vi "HistoryGraph.vi"() -> ()   [LabVIEW 2016, in "PCM MenuVIPanelSplit.lvclass"]
uses:
  PCM MenuVIPanelSplit.lvclass
  PanelSplitToolkit/PanelObject/PanelObject.lvclass
  PanelSplitToolkit/QueueManager.llb/Remove.vi
  <vilib>/Utility/error.llb/DialogType.ctl
  PanelSplitToolkit/PanelDataNode/PanelDataNode.lvclass
  PanelSplitToolkit/QueueManager.llb/Insert.vi
  PanelSplitToolkit/QueueManager.llb/CreatQueue.vi
  PanelSplitToolkit/QueueManager.llb/Destroy.vi
  <vilib>/measure/NI_MAPro.lvlib
  <vilib>/measure/maspectr.llb/FFT Spectrum (Mag-Phase) for 1 Chan.vi
  <vilib>/measure/maspectr.llb/FFT Power Spectrum and PSD for 1 Chan.vi
  <vilib>/measure/NI_MABase.lvlib
  <vilib>/Analysis/4window.llb/windowTd.ctl
  <vilib>/Analysis/NI_AALPro.lvlib
  Display Mode.ctl
  PCM PanelSplit.lvclass
  Display Config.ctl
  <vilib>/Utility/miscctls.llb/LVRangeTypeDef.ctl
panel:
  in  "Node*":refnum<data-value>
  out "波形图":waveform(dbl)[](graph)
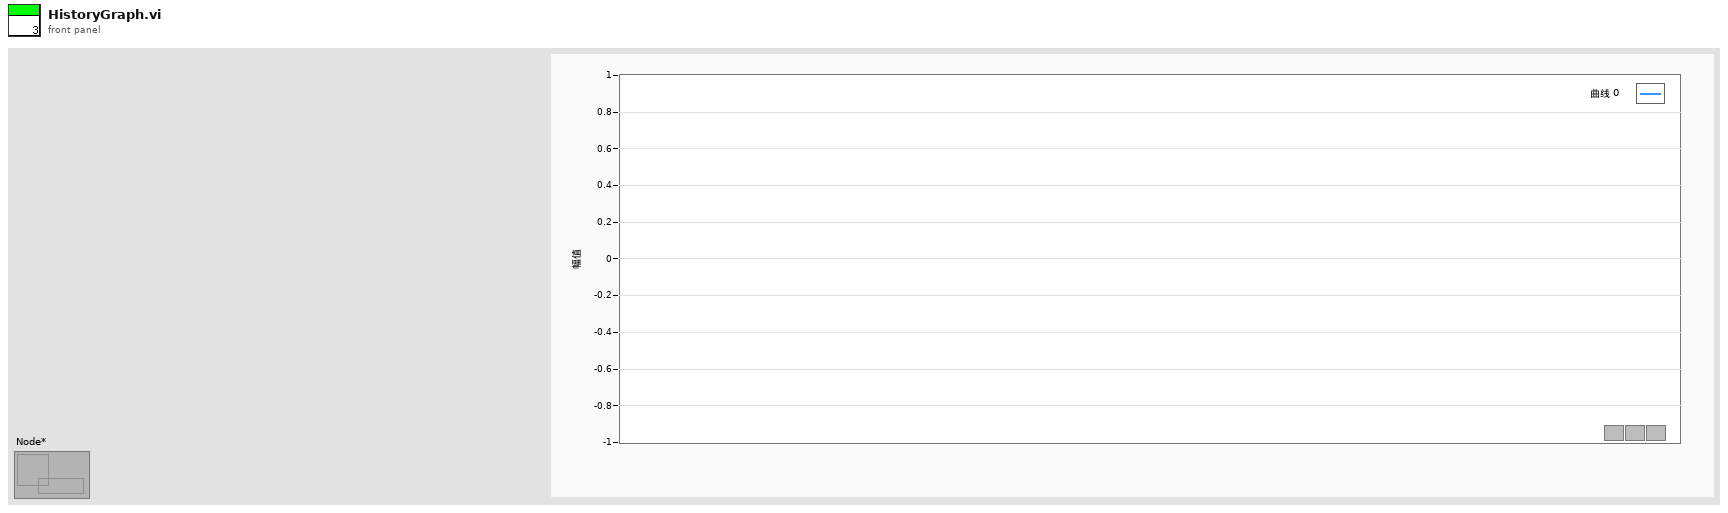
[diagram p1: front panel]
types:
  T1 = cluster{"Name":string, "Color":u32, "Style":u8, "Point Style":u8, "Name Visible":bool, "Allow Drag":bool, "Annotation Mode":u32, "Plot":i32, "Index":i32, "Position":cluster{"X":dbl, "Y":dbl}, "X Scale":u32, "Y Scale":u32, "Show Arrow":bool, "Lock Name":bool, "Plot Area":i32, "Label Offset":cluster{"X":dbl, "Y":dbl}}
  T2 = typedef "PCM PanelSplit.lvclass/Display Config.ctl" = cluster{"Display Mode":T3, "ChTag[]":string[], "window":T4, "Range":T5}
  T3 = typedef "PCM PanelSplit.lvclass/Display Mode.ctl" = enum16{"时域", "频谱", "功率谱"}
  T4 = typedef "NI_AALPro.lvlib/windowTd.ctl" = u32
  T5 = typedef "LVRangeTypeDef.ctl" = cluster{"Minimum":dbl, "Maximum":dbl, "Increment":dbl, "Minor Increment":dbl, "Start":dbl}
  T6 = cluster{"error":errorcluster, "LocalQ":cluster{"LQName":string, "LQEvent":string, "LQData":variant}, "HighQ":cluster{"HQName":string, "HQEvent":string, "HQData":variant}, "Display Config":T2, "波形图表":refnum<vi>, "波形图":refnum<vi>}
  T7 = typedef "DialogType.ctl" = u16
  T8 = typedef "Analysis Parameters.ctl" = cluster{"Enable":cluster{"Wave":bool, "Filter":bool, "FFT":bool, "Power":bool, "Shock":bool}, "IIR Parameter":T9, "FFT Parameters":T10, "Power Parameters":T12, "Shock Parameter ":T13}
  T9 = typedef "IIR Parameter.ctl" = cluster{"Filter Type":u16, "Filter Topology":u16, "Order":u32, "Lower Cut-Off":dbl, "Upper Cut-Off":dbl}
  T10 = typedef "FFT Parameters.ctl" = cluster{"window":T11, "frequency range":cluster{"start frequency":dbl, "stop frequency":dbl}, "view":cluster{"dB On (T)":bool, "unwrap phase (F)":bool, "convert to degree (T)":bool}, "averaging parameters":cluster{"averaging mode":enum16{"No averaging", "Vector averaging", "RMS averaging", "Peak hold"}, "weighting mode":enum16{"Linear", "Exponential"}, "number of averages":u32, "linear mode":enum16{"One shot", "Auto restart"}}}
  T11 = typedef "svc_Window.ctl" = u32
  T12 = typedef "Power Parameters.ctl" = cluster{"window":T11, "frequency range":cluster{"start frequency":dbl, "stop frequency":dbl}, "dB On (T)":bool, "averaging parameters":cluster{"averaging mode":enum16{"No averaging", "Vector averaging", "RMS averaging", "Peak hold"}, "weighting mode":enum16{"Linear", "Exponential"}, "number of averages":u32, "linear mode":enum16{"One shot", "Auto restart"}}}
  T13 = typedef "Shock Parameter.ctl" = cluster{"frequency range":cluster{"low frequency [Hz]":dbl, "high frequency [Hz]":dbl, "frequencies / octave":i32}, "model":i32, "critical damping factor":dbl, "preprocessing settings":cluster{"lowpass filter On ? (F)":bool, "lowpass cutoff frequency [Hz]":dbl, "remove DC ? (F)":bool}, "displacement units":i32, "maximum value type":i32, "pulse duration [ms]":dbl}
  T14 = cluster{"Name":string, "Color":u32, "Style":u8, "Point Style":u8, "Name Visible":bool, "Allow Drag":bool, "Annotation Mode":u32, "Plot":i32, "Index":i32, "Position":cluster{"X":dbl, "Y":dbl}, "X Scale":u32, "Y Scale":u32, "Show Arrow":bool, "Lock Name":bool, "Plot Area":i32, "Label Offset":cluster{"X":dbl, "Y":dbl}}[]
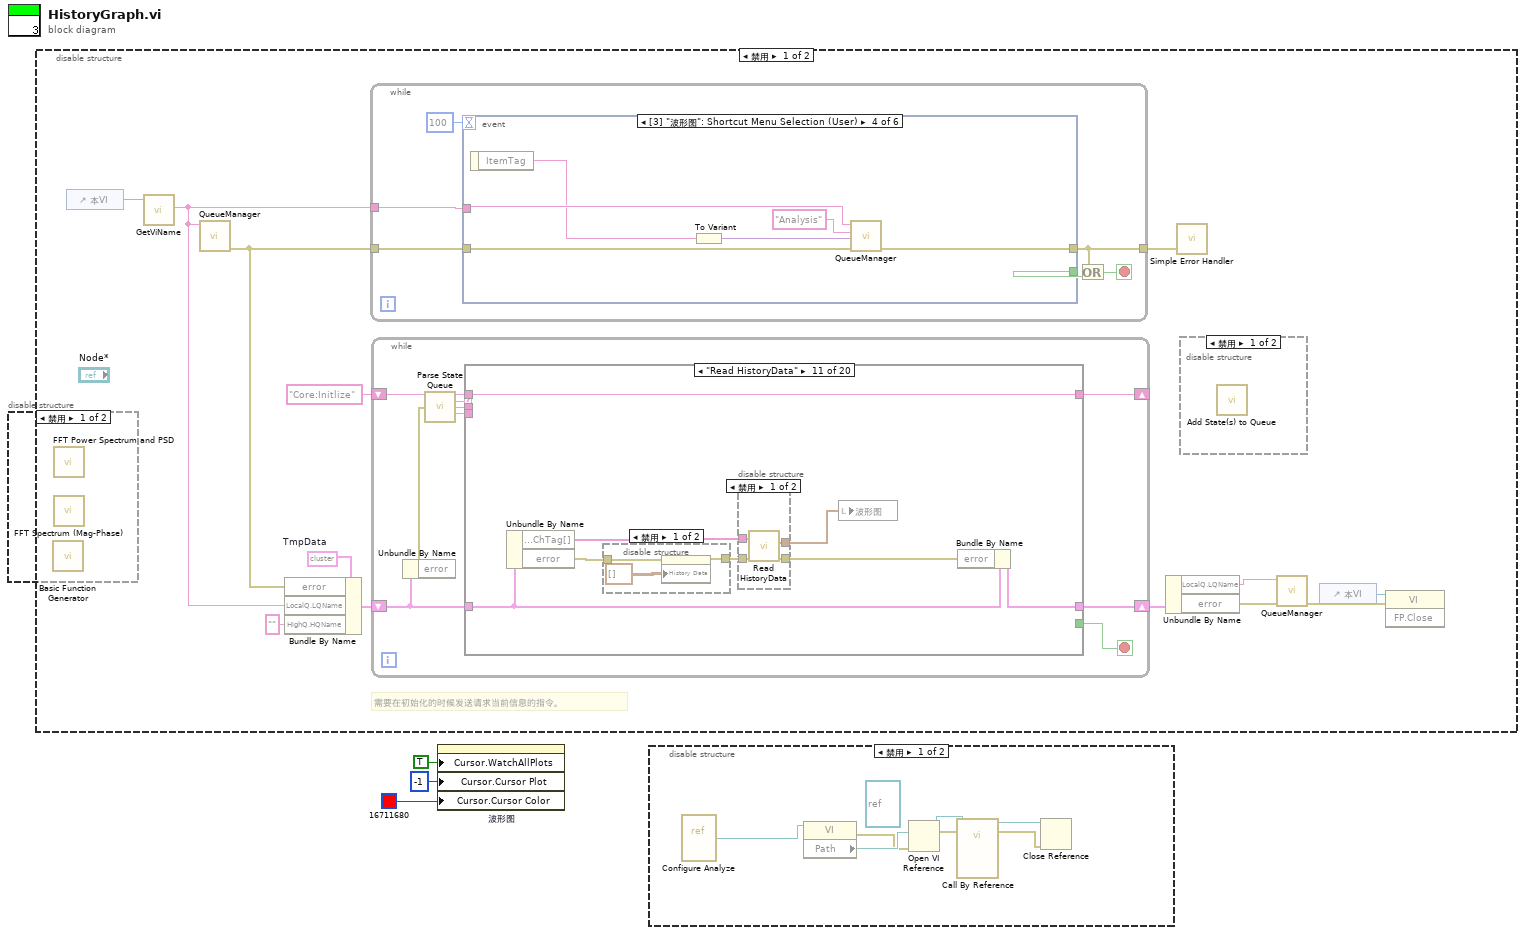
[diagram p0: block diagram]
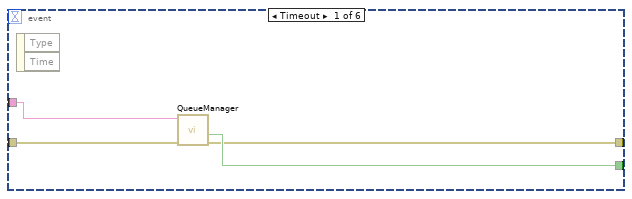
[diagram p3: hidden frame]
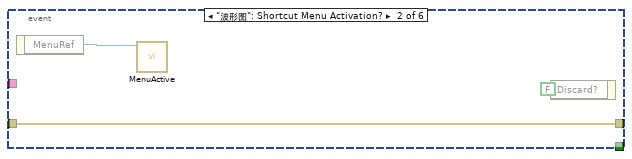
[diagram p4: hidden frame]
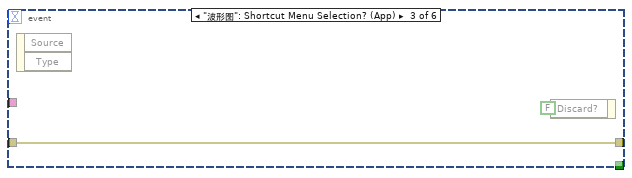
[diagram p5: hidden frame]
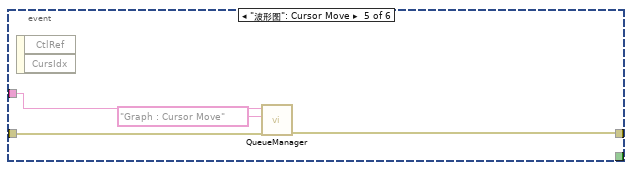
[diagram p6: hidden frame]
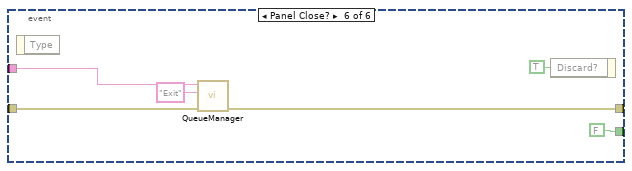
[diagram p7: hidden frame]
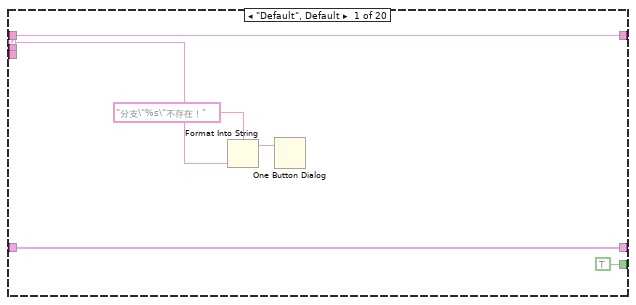
[diagram p8: hidden frame]
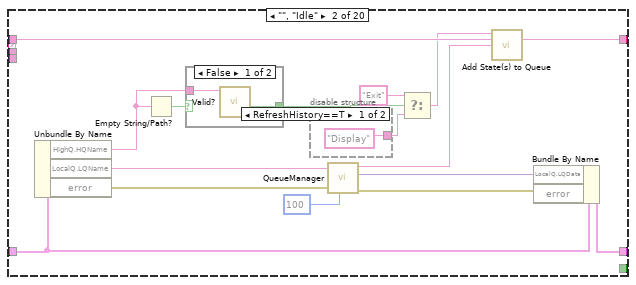
[diagram p9: hidden frame]
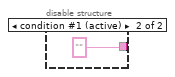
[diagram p10: hidden frame]
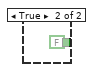
[diagram p11: hidden frame]
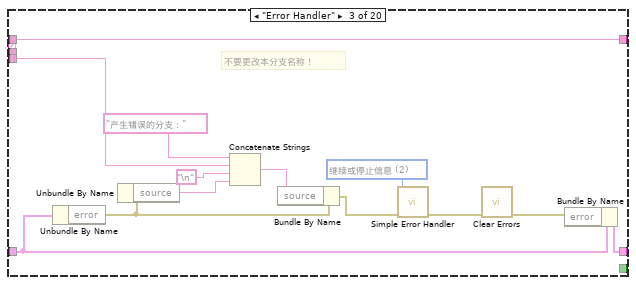
[diagram p12: hidden frame]
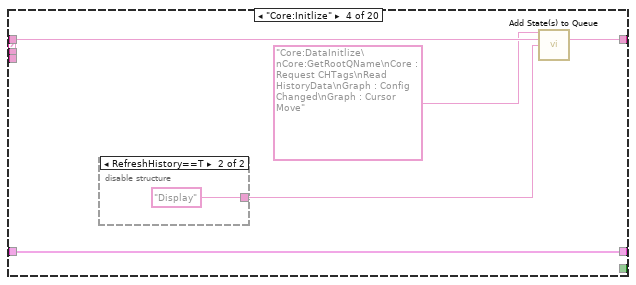
[diagram p13: hidden frame]
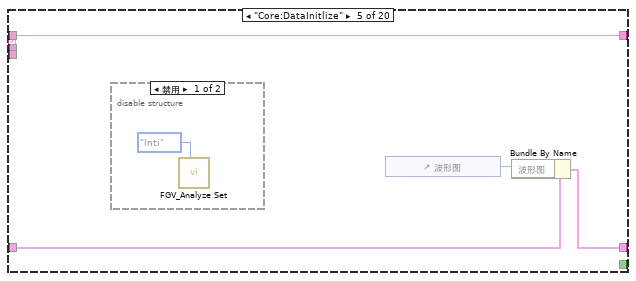
[diagram p15: hidden frame]
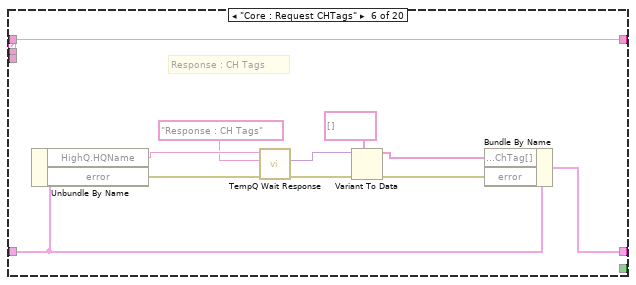
[diagram p17: hidden frame]
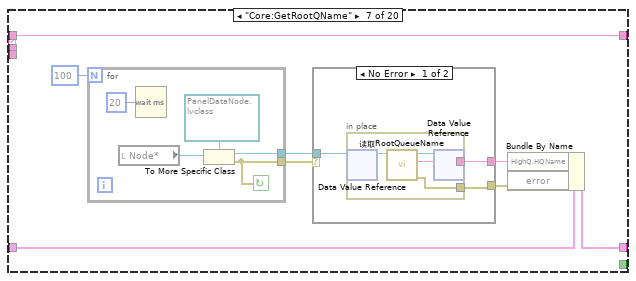
[diagram p18: hidden frame]
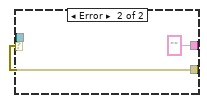
[diagram p19: hidden frame]
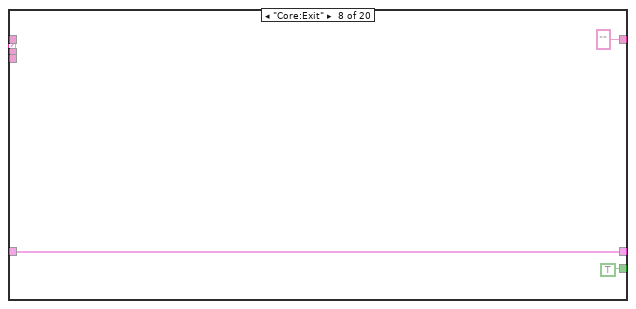
[diagram p20: hidden frame]
diagram:
  n1 = disable-structure shown="禁用" {
    frame Disabled {
      w12 = T6 {"error"={"status"=FALSE, "code"=0, "source"=""}, "LocalQ"={"LQName"="", "LQEvent"="", "LQData"=variant}, "HighQ"={"HQName"="", "HQEvent"="", "HQData"=variant}, "Display Config"={"Display Mode"=enum."时域", "ChTag[]"=[], "window"=0, "Range"={"Minimum"=0.0, "Maximum"=0.0, "Increment"=0.0, "Minor Increment"=0.0, "Start"=0.0}}, "波形图表"=refnum, "波形图"=refnum}  # TmpData
      # "需要在初始化的时候发送请求当前信息的指令。"
      n2 = disable-structure shown="禁用" {
        frame Disabled {
          n3 = call <vilib>:"Basic Function Generator.vi"() -> ()  [unwired: 9 in, 3 out]
          n4 = call-poly <vilib>:"FFT Power Spectrum and PSD.vi"() -> ()  [unwired: 8 in, 4 out]
          n5 = call-poly <vilib>:"FFT Spectrum (Mag-Phase).vi"() -> ()  [unwired: 7 in, 5 out]
        }
        frame Enabled {
        }
      }
      n6 = control-ref of="本VI"() -> (w6:refnum<vi>)
      n7 = call "GetViName.vi"("VI*"=w6) -> ("VI Name"=w7:string)  [unwired: 9 in, 1 out]
      n8 = call-poly "QueueManager.vi"("QueueName"=w7) -> ("error out"=w9:errorcluster)  [unwired: 9 in, 1 out]
      n9 = Bundle By Name(cluster=w12, "error"=w9, "LocalQ.LQName"=w7, "HighQ.HQName"="" ("Caller")) -> (w11:T6)
      n10 = while {
        tunnel: w9 -> [w21]
        tunnel: w7 -> [w22]
        tunnel: [w18] -> w13
        stop <- w19 stop-if-true
        n11 = event shown="[3] \"波形图\": Shortcut Menu Selection (User)" {
          selector: _ -> [_ _ _ _ _ _]
          dyn-events: _ -> [_ _ _ _ _ _]
          timeout: 100 -> [_ _ _ _ _ _]
          tunnel: [w24 _ _ _ _ FALSE] -> w20
          tunnel: w22 -> [w26 _ _ w34 w39 w46]
          tunnel: w21 -> [w25 w28 w30 w36 w41 w45]
          tunnel: [w23 w28 w30 w35 w40 w44] -> w18
          event Timeout {
            n12 = event-data() -> ()  [unwired: 1 in, 2 out]
            n13 = call-poly "QueueManager.vi"("error in (no error)"=w25, "Queue Name(unamed)"=w26) -> ("error out"=w23:errorcluster, "Not Exist?"=w24:bool)  [unwired: 8 in]
          }
          event "波形图": Shortcut Menu Activation? {
            n14 = event-data() -> ("MenuRef"=w27:refnum<k9>)  [unwired: 1 in]
            n15 = call "MenuActive.vi"("菜单引用"=w27) -> ()  [unwired: 11 in]
            n16 = event-data("Discard?"=FALSE ("放弃？")) -> ()  [unwired: 1 in, 1 out]
          }
          event "波形图": Shortcut Menu Selection? (App) {
            n17 = event-data() -> ()  [unwired: 1 in, 2 out]
            n18 = event-data("Discard?"=FALSE ("放弃？")) -> ()  [unwired: 1 in, 1 out]
          }
          event "波形图": Shortcut Menu Selection (User) {
            n19 = event-data() -> ("ItemTag"=w33:string)  [unwired: 1 in]
            n20 = To Variant(anything=w33) -> (Variant=w32:variant)
            n21 = call-poly "QueueManager.vi"("error in"=w36, "Data"=w32, "Event"="Analysis", "QueueName"=w34) -> ("error out"=w35:errorcluster)  [unwired: 6 in, 1 out]
          }
          event "波形图": Cursor Move {
            n22 = event-data() -> ()  [unwired: 1 in, 2 out]
            n23 = call-poly "QueueManager.vi"("error in"=w41, "Event"="Graph : Cursor Move", "QueueName"=w39) -> ("error out"=w40:errorcluster)  [unwired: 7 in, 1 out]
          }
          event Panel Close? {
            n24 = event-data() -> ()  [unwired: 1 in, 1 out]
            n25 = call-poly "QueueManager.vi"("error in"=w45, "Event"="Exit", "QueueName"=w46) -> ("error out"=w44:errorcluster)  [unwired: 7 in, 1 out]
            n26 = event-data("Discard?"=TRUE ("放弃？")) -> ()  [unwired: 1 in, 1 out]
          }
        }
        n27 = Or(x=w18, y=w20) -> (x .or. y?=w19:bool)
      }
      n28 = while {
        shift-right: [w51] -> w14
        shift-left: w11 -> [w52]
        shift-right: [w50] -> _
        shift-left: "Core:Initlize" -> [w57]
        stop <- w54 stop-if-true
        n29 = Unbundle By Name(w52) -> ("error"=w53:errorcluster)
        n30 = call "Parse State Queue.vi"("State Queue"=w57, "Error In (no error)"=w53) -> ("Remaining States"=w56:string, "Current State"=w55:string, "Arguments"=w49:string, "PreState"=w48:string)  [unwired: 10 in]
        n31 = case shown="\"Read HistoryData\"" w55 {
          selector: w55 -> [w61 _ _ _ _ _ _ _ _ _ _ _ _ _ _ _ _ _ _ _]
          tunnel: w56 -> [w62 w76 w97 w101 w107 w119 w127 _ _ w148 w158 w175 w184 w205 w226 w228 w232 w242 w252 w260]
          tunnel: w49 -> [_ _ _ _ _ _ _ _ _ _ _ _ _ _ _ _ _ _ _ _]
          tunnel: [TRUE _ _ _ _ _ _ TRUE FALSE FALSE _ _ _ _ _ _ _ _ _ _] -> w54
          tunnel: w52 -> [w63 w73 w94 w102 w106 w116 w123 w143 w146 w149 w157 w174 w183 w204 w227 w229 w236 w246 w256 w261]
          tunnel: [w63 w78 w93 w102 w105 w118 w122 w143 w146 w149 w156 w173 w182 w204 w227 w229 w235 w245 w255 w261] -> w51
          tunnel: [w62 w75 w97 w100 w107 w119 w127 "" ("Remaining States") "Core:Exit" ("Remaining States") w148 w158 w175 w184 w205 w226 w228 w231 w241 w251 w260] -> w50
          tunnel: w48 -> [_ _ w91 _ _ _ _ _ _ _ _ _ _ _ _ _ _ _ _ _]
          frame "Default", Default {
            n32 = Format Into String(format string="分支\"%s\"不存在！" ("格式字符串"), w61) -> (resulting string=w60:string)  [unwired: 2 in, 1 out]
            n33 = One Button Dialog(message=w60) -> ()  [unwired: 1 in, 1 out]
          }
          frame "", "Idle" {
            n34 = Unbundle By Name(w73) -> ("HighQ.HQName"=w67:string, "LocalQ.LQName"=w72:string, "error"=w71:errorcluster)
            n35 = Empty String/Path?(string/path=w67) -> (empty?=w70:bool)
            n36 = case shown="False" w70 {
              tunnel: [w83 FALSE ("Not Exist?")] -> w69
              tunnel: w67 -> [w82 _]
              frame False {
                n37 = call "Valid?.vi"("Queue Name(unamed)"=w82) -> ("Not Exist?"=w83:bool)  [unwired: 9 in, 1 out]
              }
              frame True {
              }
            }
            n38 = disable-structure shown="RefreshHistory==T" {
              disable-tunnel: ["Display" ("f") "" ("f")] -> w64
              frame condition #0 {
              }
              frame condition #1 (active) {
              }
            }
            n39 = call-poly "QueueManager.vi"("Time out(-1)"=100, "error in (no error)"=w71, "Queue Name"=w72) -> ("error out"=w79:errorcluster, "Data"=w77:variant, "Event"=w66:string)  [unwired: 5 in, 1 out]
            n40 = Select(t="Exit" ("Event"), s=w69, f=w64) -> (s? t:f=w65:string)
            n41 = call "Add State(s) to Queue.vi"("State(s) in Front (\"\")"=w65, "State(s) in (\"\")"=w76, "State(s) at Back (\"\")"=w66) -> ("States Out"=w75:string)  [unwired: 12 in]
            n42 = Bundle By Name(cluster=w73, "LocalQ.LQData"=w77, "error"=w79) -> (w78:T6)
          }
          frame "Error Handler" {
            w92 = T7 2 items=["无对话框", "确定信息", "继续或停止信息", "确定信息＋警告", "继续/停止+警告"] ("type of dialog (OK msg:1)")
            # "不要更改本分支名称！"
            n43 = Unbundle By Name(w94) -> ("error"=w86:errorcluster)
            n44 = Unbundle By Name(w86) -> ("source"=w89:string)
            n45 = Concatenate Strings("产生错误的分支：" ("字符串"), w91, "\n", w89) -> (w87:string)
            n46 = Bundle By Name(cluster=w86, "source"=w87) -> (w85:errorcluster)
            n47 = call <vilib>:"Simple Error Handler.vi"("type of dialog (OK msg:1)"=w92, "error in (no error)"=w85) -> ("error out"=w95:errorcluster)  [unwired: 3 in, 4 out]
            n48 = call <vilib>:"Clear Errors.vi"("error in (no error)"=w95) -> ("error out"=w96:errorcluster)  [unwired: 5 in, 1 out]
            n49 = Bundle By Name(cluster=w94, "error"=w96) -> (w93:T6)
          }
          frame "Core:Initlize" {
            n50 = disable-structure shown="RefreshHistory==T" {
              disable-tunnel: [_ "Display"] -> w98
              frame condition #0 (active) {
              }
              frame condition #1 {
              }
            }
            n51 = call "Add State(s) to Queue.vi"("State(s) in Front (\"\")"="Core:DataInitlize\nCore:GetRootQName\nCore : Request CHTags\nRead HistoryData\nGraph : Config Changed\nGraph : Cursor Move" ("State(s) at Back (\"\")"), "State(s) in (\"\")"=w101, "State(s) at Back (\"\")"=w98) -> ("States Out"=w100:string)  [unwired: 12 in]
          }
          frame "Core:DataInitlize" {
            n52 = disable-structure shown="禁用" {
              frame Disabled {
                n53 = call "FGV_Analyze Set.vi"("Action"=enum16{"Inti", "Write", "Read"}."Inti") -> ()  [unwired: 9 in, 2 out]
              }
              frame Enabled {
              }
            }
            n54 = control-ref of="波形图"() -> (w104:refnum<vi>)
            n55 = Bundle By Name(cluster=w106, "波形图"=w104) -> (w105:T6)
          }
          frame "Core : Request CHTags" {
            # "Response : CH Tags"
            n56 = Unbundle By Name(w116) -> ("HighQ.HQName"=w114:string, "error"=w115:errorcluster)
            n57 = call "TempQ Wait Response.vi"("error in"=w115, "Event"="Response : CH Tags", "TargetQName"=w114) -> ("error out"=w112:errorcluster, "Data"=w117:variant)  [unwired: 5 in, 2 out]
            n58 = Variant To Data(error in=w112, type=string[] [] ("Display Config.Display CH Tag[]"), Variant=w117) -> (data=w109:string[], error out=w111:errorcluster)
            n59 = Bundle By Name(cluster=w116, "Display Config.ChTag[]"=w109, "error"=w111) -> (w118:T6)
          }
          frame "Core:GetRootQName" {
            n60 = for {
              N: 100 -> [_]
              tunnel: [w139] -> w124
              tunnel: [w138] -> w121
              stop <- w138 continue-if-true
              n61 = local read "Node*"() -> (w141:refnum<data-value>)
              n62 = Wait (ms)(milliseconds to wait=u32 20 ("等待时间（毫秒）")) -> ()  [unwired: 1 out]
              n63 = To More Specific Class(target class=refnum<data-value> refnum ("Node*"), reference=w141) -> (specific class reference=w139:refnum<data-value>, error out=w138:errorcluster)  [unwired: 1 in]
            }
            n64 = case shown="No Error" w121 {
              selector: w121 -> [_ w136]
              tunnel: [w128 w136] -> w126
              tunnel: [w130 "" ("RootQueueName")] -> w125
              tunnel: w124 -> [w129 _]
              frame No Error {
                n65 = in-place {
                  in-place-border: [w132] -> w130
                  in-place-border: [w131] -> w128
                  n66 = in-place-dvr #1(w129) -> (w134:refnum<class "PanelDataNode.lvclass">)  [unwired: 1 out]
                  n67 = call "读取RootQueueName.vi"("PanelDataNode输入"=w134) -> ("error out"=w131:errorcluster, "RootQueueName"=w132:string, "PanelDataNode输出"=w133:refnum<class "PanelDataNode.lvclass">)  [unwired: 8 in]
                  n68 = in-place-dvr #1(w133) -> ()  [unwired: 2 out]
                }
              }
              frame Error {
              }
            }
            n69 = Bundle By Name(cluster=w123, "HighQ.HQName"=w125, "error"=w126) -> (w122:T6)
          }
          frame "Core:Exit" {
          }
          frame "Exit" {
          }
          frame "-----User Event------" {
          }
          frame "Read HistoryData" {
            n70 = Unbundle By Name(w157) -> ("Display Config.ChTag[]"=w153:string[], "error"=w155:errorcluster)
            n71 = disable-structure shown="禁用" {
              disable-tunnel: w155 -> [w165 w166]
              disable-tunnel: [w164 w166] -> w154
              frame Disabled {
                n72 = property on="波形图" class="WFGraph (strict)"(error in=w165, "History Data"=waveform(dbl)[][] [] ("历史数据")) -> (error out=w164:errorcluster)  [unwired: 1 in, 1 out]
              }
              frame Enabled {
              }
            }
            n73 = disable-structure shown="禁用" {
              disable-tunnel: w154 -> [w162 _]
              disable-tunnel: w153 -> [w161 _]
              disable-tunnel: [w160 _] -> w152
              disable-tunnel: [w159 _] -> w151
              frame Disabled {
                n74 = call "Read HistoryData.vi"("error in"=w162, "Channel Tag[]"=w161) -> ("error out"=w159:errorcluster, "Waveform"=w160:waveform(dbl)[])  [unwired: 8 in]
              }
              frame Enabled {
              }
            }
            n75 = local write "波形图"(w152) -> ()
            n76 = Bundle By Name(cluster=w157, "error"=w151) -> (w156:T6)
          }
          frame "Display" {
            n77 = Unbundle By Name(w174) -> ("Display Config.ChTag[]"=w171:string[], "error"=w170:errorcluster)
            n78 = Wait (ms)(milliseconds to wait=u32 150 ("等待时间（毫秒）")) -> ()  [unwired: 1 out]
            n79 = call "DataQ GetWaveform.vi"("error in"=w170, "ChannelTag[]"=w171) -> ("error out"=w169:errorcluster, "Valid?"=w168:bool, "Waveform"=w167:waveform(dbl)[])  [unwired: 7 in]
            n80 = case shown="True" w168 {
              tunnel: w167 -> [_ w177]
              frame False {
              }
              frame True {
                n81 = for {
                  tunnel: w177 -> [w178] mode=indexing
                  tunnel: [w179] -> w176 mode=indexing
                  n82 = Unbundle By Name(w178) -> ("attributes"=w181:variant, "t0"=w180:timestamp)
                  n83 = call "BuildIndexWaveform.vi"("t0"=w180, "attributes"=w181) -> ("输出波形"=w179:waveform(dbl))  [unwired: 9 in]
                }
                "波形图" <- w176
              }
            }
            n84 = Bundle By Name(cluster=w174, "error"=w169) -> (w173:T6)
          }
          frame "Analysis" {
            n85 = disable-structure shown="启用" {
              disable-tunnel: w183 -> [w188 _]
              disable-tunnel: [w187 _] -> w182
              frame Disabled {
                n86 = Unbundle By Name(w188) -> ("Display Config.ChTag[]"=w190:string[], "LocalQ.LQName"=w186:string, "LocalQ.LQData"=w195:variant, "error"=w196:errorcluster)
                n87 = control-ref of="波形图"() -> (w191:refnum<vi>)
                n88 = Variant To Data(error in=w196, type=w186, Variant=w195) -> (data=w192:string, error out=w194:errorcluster)
                n89 = call "Get Select Data.vi"("Channel Tag[]"=w190, "波形图"=w191) -> ("Data"=w193:waveform(sgl)[])  [unwired: 9 in]
                n90 = call "Configure Analyze for History.vi"("Q-Caller"=w186) -> ("Analysis Parameters"=w185:T8)  [unwired: 10 in]
                n91 = call "Detail FFT.vi"("error in (no error)"=w194, "Analysis Parameters"=w185, "Waveform"=w193, "Type"=w192) -> ("error out"=w189:errorcluster)  [unwired: 7 in]
                n92 = Bundle By Name(cluster=w188, "error"=w189) -> (w187:T6)
              }
              frame Enabled {
              }
            }
          }
          frame "Graph : Config Changed" {
            # "更改曲线名、Y标签，是否需要？"
            n93 = Unbundle By Name(w204) -> ("波形图"=w199:refnum<vi>, "Display Config.ChTag[]"=w202:string[])
            n94 = call "Convert Channel Tag And Name.vi"("Direction"=enum16{"Tag to Name", "Name to Tag"}."Tag to Name", "String[] in"=w202) -> ("String[] out"=w198:string[])  [unwired: 8 in, 1 out]
            n95 = Array Size(array=w198) -> (size(s)=w200:i32)
            n96 = property on="属性节点" class="WFGraph (严格)"(reference=w199, "LegPlotMin"=w200, "LegNumRows"=w200) -> (reference out=w201:refnum<vi>, error out=w197:errorcluster)  [unwired: 1 in]
            n97 = for {
              tunnel: w201 -> [w213]
              tunnel: w198 -> [w210] mode=indexing
              tunnel: [w209] -> _
              tunnel: w197 -> [w206]
              i -> [w212]
              n98 = Concatenate Strings(w210, " - " ("格式字符串"), "历史" ("格式字符串")) -> (w208:string)
              n99 = property class="WFGraph (严格)"(reference=w213, error in=w206, "Active Plot"=w212, "Plot.Plot Name"=w208) -> (error out=w209:errorcluster)  [unwired: 1 out]
            }
          }
          frame "Graph : Cursor Move" {
            n100 = property on="波形图" class="WFGraph (strict)"() -> ("Cursor.Cursor X"=w217:dbl, "Cursor.Cursor Y"=w221:dbl)  [unwired: 2 in, 2 out]
            n101 = To Time Stamp(1:w217) -> (0:w216:timestamp)
            n102 = Format Date/Time String(time format string (%c)="%H:%M:%S" ("时间格式字符串(%c)"), seconds (now)=w216) -> (date/time string=w215:string)  [unwired: 1 in]
            n103 = Format Into String(format string="(%s , %.2f)" ("格式字符串"), w215, w221) -> (resulting string=w223:string)  [unwired: 2 in, 1 out]
            n104 = Bundle By Name(cluster=T1 {"Name"="", "Color"=0, "Style"=0, "Point Style"=0, "Name Visible"=FALSE, "Allow Drag"=FALSE, "Annotation Mode"=0, "Plot"=0, "Index"=0, "Position"={"X"=0.0, "Y"=0.0}, "X Scale"=0, "Y Scale"=0, "Show Arrow"=FALSE, "Lock Name"=FALSE, "Plot Area"=0, "Label Offset"={"X"=0.0, "Y"=0.0}}, "Name"=w223, "Color"=u32 0, "Name Visible"=TRUE, "Position.X"=w217, "Position.Y"=w221) -> (w219:T1)
            n105 = Build Array(w219) -> (w218:T14)
            n106 = property on="波形图" class="WFGraph (strict)"("AnntList"=w218) -> ()  [unwired: 2 in, 2 out]
          }
          frame "---Communication---" {
          }
          frame "Rec : Channel Changed" {
            n107 = Unbundle By Name(w236) -> ("Display Config.ChTag[]"=w237:string[], "LocalQ.LQData"=w238:variant, "error"=w239:errorcluster)
            n108 = Variant To Data(error in=w239, type=w237, Variant=w238) -> (data=w233:string[], error out=w234:errorcluster)
            n109 = Bundle By Name(cluster=w236, "Display Config.ChTag[]"=w233, "error"=w234) -> (w235:T6)
            n110 = call "Add State(s) to Queue.vi"("State(s) in Front (\"\")"="Graph : Config Changed\nRead HistoryData", "State(s) in (\"\")"=w232) -> ("States Out"=w231:string)  [unwired: 13 in]
          }
          frame "Rec : Window Changed" {
            n111 = Unbundle By Name(w246) -> ("Display Config.window"=w247:T4, "LocalQ.LQData"=w248:variant, "error"=w249:errorcluster)
            n112 = Variant To Data(error in=w249, type=w247, Variant=w248) -> (data=w243:T4, error out=w244:errorcluster)
            n113 = Bundle By Name(cluster=w246, "Display Config.window"=w243, "error"=w244) -> (w245:T6)
            n114 = call "Add State(s) to Queue.vi"("State(s) in Front (\"\")"="Graph : Config Changed", "State(s) in (\"\")"=w242) -> ("States Out"=w241:string)  [unwired: 13 in]
          }
          frame "Rec : DisplayMode Changed" {
            n115 = Unbundle By Name(w256) -> ("Display Config.Display Mode"=w257:T3, "LocalQ.LQData"=w258:variant, "error"=w259:errorcluster)
            n116 = Variant To Data(error in=w259, type=w257, Variant=w258) -> (data=w253:T3, error out=w254:errorcluster)
            n117 = Bundle By Name(cluster=w256, "Display Config.Display Mode"=w253, "error"=w254) -> (w255:T6)
            n118 = call "Add State(s) to Queue.vi"("State(s) in (\"\")"=w252, "State(s) at Back (\"\")"="Graph : Config Changed") -> ("States Out"=w251:string)  [unwired: 13 in]
          }
          frame "Transfer : Channel Changed" {
          }
        }
      }
      n119 = Unbundle By Name(w14) -> ("LocalQ.LQName"=w10:string, "error"=w15:errorcluster)
      n120 = call <vilib>:"Simple Error Handler.vi"("error in (no error)"=w13) -> ()  [unwired: 4 in, 5 out]
      n121 = disable-structure shown="禁用" {
        frame Disabled {
          n122 = call "Add State(s) to Queue.vi"() -> ()  [unwired: 15 in, 1 out]
        }
        frame Enabled {
        }
      }
      n123 = call-poly "QueueManager.vi"("error in (no error)"=w15, "QueeuName"=w10) -> ("error out"=w4:errorcluster)  [unwired: 9 in]
      n124 = control-ref of="本VI"() -> (w5:refnum<vi>)
      n125 = invoke class="VI" method="FP.Close"(reference=w5, error in=w4) -> ()  [unwired: 1 in, 3 out]
    }
    frame Enabled {
    }
  }
  n126 = property on="波形图" class="WFGraph (strict)"("Cursor.WatchAllPlots"=TRUE ("游标.监视所有曲线"), "Cursor.Cursor Plot"=-1 ("游标.游标关联曲线"), "Cursor.Cursor Color"=u32 16711680) -> ()  [unwired: 2 in, 2 out]
  n127 = disable-structure shown="禁用" {
    frame Disabled {
      (unwired) refnum<vi> refnum
      n128 = vi-ref "Configure Analyze.vi"() -> (w268:refnum<vi>)
      n129 = property class="VI"(reference=w268) -> (error out=w262:errorcluster, "Path"=w263:path)  [unwired: 1 in, 1 out]
      n130 = Open VI Reference(vi path=w263, error in (no error)=w262) -> (vi reference=w265:refnum<vi>, error out=w264:errorcluster)  [unwired: 4 in]
      n131 = call-by-ref "?"(reference=w265, error in=w264) -> (reference out=w267:refnum<vi>, error out=w266:errorcluster)  [unwired: 11 in, 1 out]
      n132 = Close Reference(reference=w267, error in (no error)=w266) -> ()  [unwired: 1 out]
    }
    frame Enabled {
    }
  }
